vi "Write Description.vi"(8 "error in (no error)":errorcluster, 10 "description":string, 11 "Base Interface in":refnum<class "Base Interface.lvclass">) -> (0 "error out":errorcluster, 3 "Base Interface out":refnum<class "Base Interface.lvclass">)   [LabVIEW 2020, in "PV Access.lvlib" / "PV Data.lvlib" / "Base Interface.lvclass"]
uses:
  Base Interface.lvclass
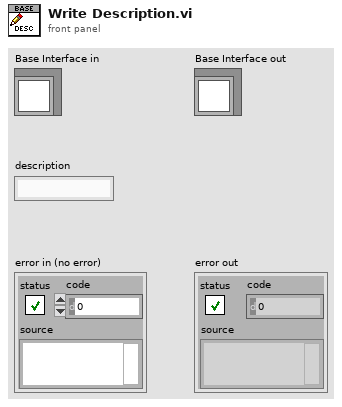
[diagram p1: front panel]
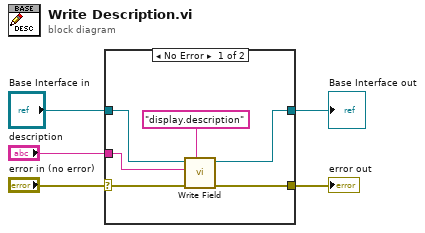
[diagram p0: block diagram]
diagram:
  n1 = case shown="No Error" "error in (no error)" {
    selector: "error in (no error)" -> [w7 w13]
    tunnel: [w8 w13] -> w4
    tunnel: [w9 w12] -> w2
    tunnel: "Base Interface in" -> [w10 w12]
    tunnel: "description" -> [w6 _]
    frame No Error {
      n2 = call-dynamic "Write Field.vi"("field"="display.description", "error in (no error)"=w7, "value"=w6, "Base Interface in"=w10) -> ("error out"=w8:errorcluster, "Base Interface out"=w9:refnum<class "Base Interface.lvclass">)  [unwired: 6 in]
    }
    frame Error {
    }
  }
  "error out" <- w4
  "Base Interface out" <- w2
